vi "Configure.vi"(8 "error in (no error)":errorcluster, 11 "Template in":refnum<class "PockelCell.lvclass">) -> (0 "error out":errorcluster, 2 "cancelled?":bool, 3 "Template out":refnum<class "PockelCell.lvclass">)   [LabVIEW 2012, in "PockelCell.lvclass"]
doc: "The configure method configures the details for the RabbitMQ connection. \n\nIn the derived class, make a call to the parent for setting these parameters."
uses:
  PockelCell.lvclass
  <vilib>/Utility/miscctls.llb/LVPointTypeDef.ctl
  <vilib>/Distrio/Murmex/Murmex/Murmex.lvclass
panel:
  in  "Samples per channel":i32
  in  "Sample rate":dbl
  in  "button:call parent":bool
  in  "button:ok":bool
  in  "button:cancel":bool
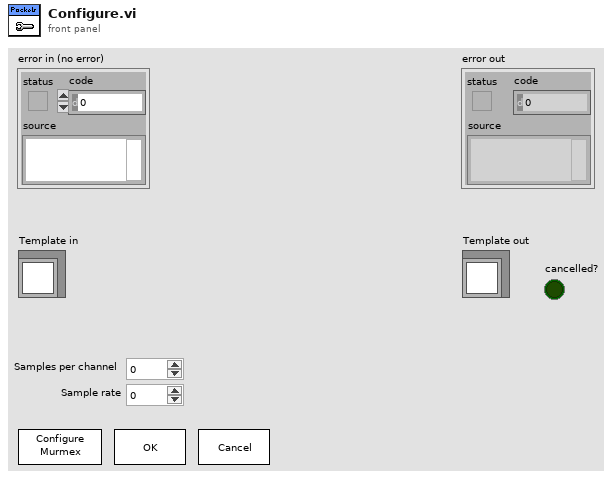
[diagram p1: front panel]
types:
  T1 = typedef "LVPointTypeDef.ctl" = cluster{"Horizontal":i16, "Vertical":i16}
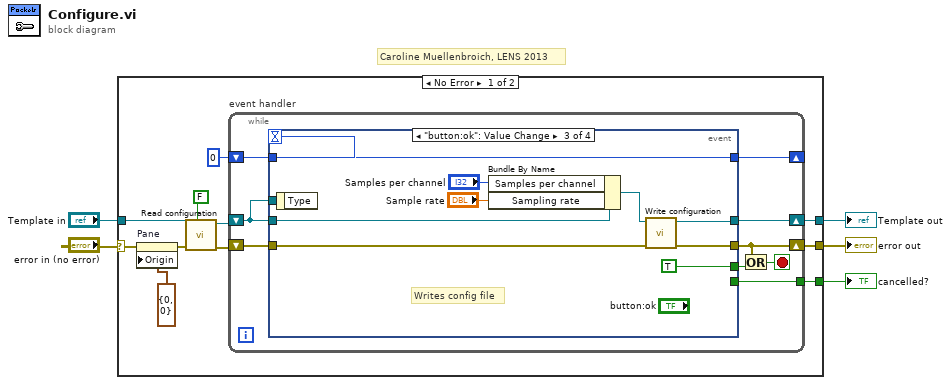
[diagram p0: block diagram]
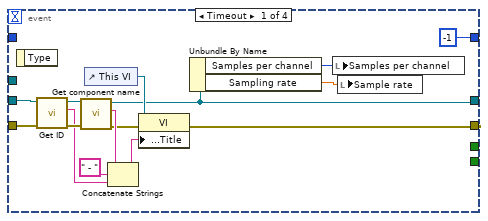
[diagram p2: hidden frame]
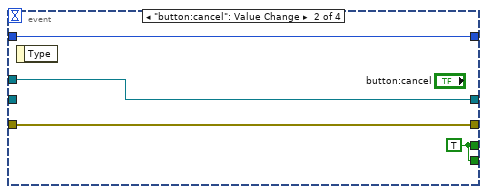
[diagram p3: hidden frame]
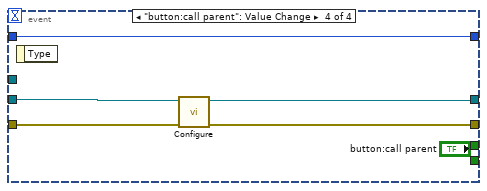
[diagram p4: hidden frame]
diagram:
  # "Caroline Muellenbroich, LENS 2013"
  n1 = case shown="No Error" "error in (no error)" {
    selector: "error in (no error)" -> [w11 w59]
    tunnel: [w16 w59] -> w5
    tunnel: [w15 _] -> w4
    tunnel: [w14 w60] -> w3
    tunnel: "Template in" -> [w8 w60]
    frame No Error {
      n2 = property on="Pane" class="Pane"(error in=w11, "Origin"=T1 {"Horizontal"=0, "Vertical"=0}) -> (error out=w10:errorcluster)  [unwired: 1 in, 1 out]
      n3 = call-dynamic "Read configuration.vi"("force loading?"=FALSE, "error in (no error)"=w10, "Template in"=w8) -> ("error out"=w9:errorcluster, "Template out"=w7:refnum<class "PockelCell.lvclass">)  [unwired: 7 in]
      n4 = while "event handler" {
        tunnel: [w25] -> w15
        shift-right: [w24] -> w14
        shift-left: w7 -> [w22]
        shift-right: [w21] -> w16
        shift-left: w9 -> [w23]
        shift-right: [w18] -> _
        shift-left: 0 -> [w17]
        stop <- w19 stop-if-true
        n5 = event shown="[2] \"button:ok\": Value Change" {
          selector: _ -> [_ _ _ _]
          dyn-events: _ -> [_ _ _ _]
          timeout: w17 -> [_ _ _ _]
          tunnel: [w31 w43 w48 w56] -> w21
          tunnel: [_ w42 _ _] -> w25
          tunnel: [w28 w44 w50 w55] -> w24
          tunnel: w23 -> [w39 w43 w49 w57]
          tunnel: w22 -> [w30 _ w52 w58]
          tunnel: w22 -> [_ w44 _ _]
          tunnel: [_ w42 TRUE ("cancelled?") _] -> w20
          tunnel: [-1 w41 w47 w54] -> w18
          tunnel: w17 -> [_ w41 w47 w54]
          event Timeout {
            n6 = event-data() -> ()  [unwired: 1 in, 1 out]
            n7 = call "Get ID.vi"("error in (no error)"=w39, "Murmex in"=w30) -> ("error out"=w38:errorcluster, "component id"=w36:string, "Murmex out"=w29:refnum<class "PockelCell.lvclass">)  [unwired: 7 in]
            n8 = call "Get component name.vi"("error in (no error)"=w38, "Murmex in"=w29) -> ("error out"=w34:errorcluster, "component name"=w35:string, "Murmex out"=w28:refnum<class "PockelCell.lvclass">)  [unwired: 7 in]
            n9 = control-ref of="This VI"() -> (w32:refnum<vi>)
            n10 = Concatenate Strings(w35, " - " ("string"), w36) -> (w33:string)
            n11 = property class="VI"(reference=w32, error in=w34, "Front Panel.Title"=w33) -> (error out=w31:errorcluster)  [unwired: 1 out]
            n12 = Unbundle By Name(w28) -> ("Samples per channel"=w27:i32, "Sampling rate"=w26:dbl)
            n13 = local write "Samples per channel"(w27) -> ()
            n14 = local write "Sample rate"(w26) -> ()
          }
          event "button:cancel": Value Change {
            w42 = TRUE ("cancelled?")
            n15 = event-data() -> ()  [unwired: 1 in, 1 out]
          }
          event "button:ok": Value Change {
            # "Writes config file"
            n16 = event-data() -> ()  [unwired: 1 in, 1 out]
            n17 = Bundle By Name(cluster=w52, "Samples per channel"="Samples per channel", "Sampling rate"="Sample rate") -> (w51:refnum<class "PockelCell.lvclass">)
            n18 = call-dynamic "Write configuration.vi"("error in (no error)"=w49, "Template in"=w51) -> ("error out"=w48:errorcluster, "Template out"=w50:refnum<class "PockelCell.lvclass">)  [unwired: 8 in]
          }
          event "button:call parent": Value Change {
            n19 = event-data() -> ()  [unwired: 1 in, 1 out]
            n20 = call-parent "Configure.vi"("error in (no error)"=w57, "Murmex in"=w58) -> ("error out"=w56:errorcluster, "Murmex out"=w55:refnum<class "PockelCell.lvclass">)  [unwired: 7 in, 1 out]
          }
        }
        n21 = Or(x=w21, y=w20) -> (x .or. y?=w19:bool)
      }
    }
    frame Error {
    }
  }
  "error out" <- w5
  "Template out" <- w3
  "cancelled?" <- w4
